vi "New Process.vi"(8 "error in (no error)":errorcluster, 10 "Init options":T1={"UI visible?"=TRUE, "Update rate (ms)"=250, "visible sidebar?"=TRUE, "time to plot (init)"=600.0, "time to plot (max)"=inf, "config file start path"=path ""} {"time to plot (init)" format="%<%H:%M:%S>t"}, 11 "BluePlotHandle in":refnum<class "BluePlotHandle.lvclass">) -> (0 "error out":errorcluster, 2 "VI ref":refnum<vi>, 3 "BluePlotHandle out":refnum<class "BluePlotHandle.lvclass">)   [LabVIEW 2021, in "BluePlot.lvlib" / "BluePlotHandle.lvclass"]
doc: "This will launch a new asynchronous plot instance.\n\n<B>BluePlotHandle in\n</B>This needs to be a user-created object which has dynamic dispatch overrides for satisfying the framework of the package.\n\n<B>Init options</B>\nOptional arguments for affecting the bootup behavior of the plot instance.\nUI Visibile --> Is the UI visible? If no, then the plots are not updated.\nUpdate rate (ms) --> refresh rate of the plots\nvisible sidebar? --> Is the sidebar displaing channel names visible?\ntime to plot (init) --> initial value for the time-to-plot control\ntime to plot (max) --> max allowed entry value for the time-to-plot control\n\n<B>VI ref</B>\nThis output is a reference to the launched plot instance.\nYou are able to insert this into a subpanel, or just open the front panel directly."
uses:
  BluePlotHandle.lvclass
  SubVIs/Init Options.ctl
  TypeDefs/BlueMultiPlot Inputs.ctl
  BluePlot.lvlib
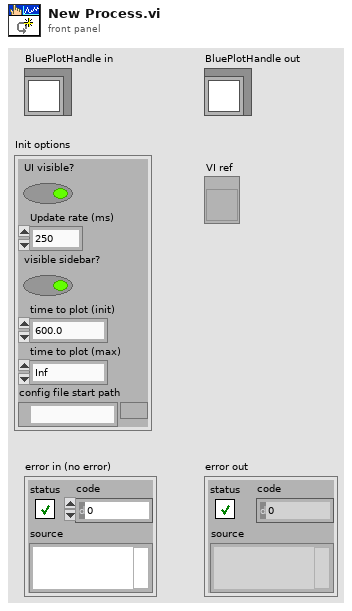
[diagram p1: front panel]
types:
  T1 = typedef "BluePlot.lvlib/BluePlotHandle.lvclass/Init Options.ctl" = cluster{"UI visible?":bool, "Update rate (ms)":u32, "visible sidebar?":bool, "time to plot (init)":dbl, "time to plot (max)":dbl, "config file start path":path}
  T2 = typedef "BluePlot.lvlib/BlueMultiPlot Inputs.ctl" = cluster{"plot menu":string[], "UE: ItemTag":refnum<user-event>}
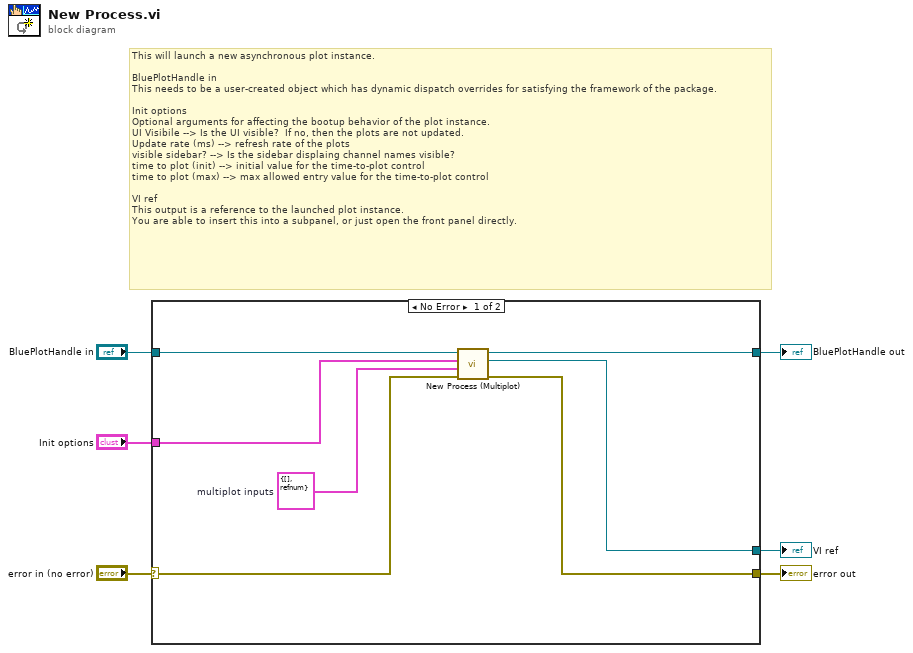
[diagram p0: block diagram]
diagram:
  # "This will launch a new asynchronous plot instance.\n\nBluePlotHandle in\nThis needs to be a user-created object which has dynamic dispatch overrides for satisfying the framework of the package.\n\nInit options\nOptional arguments for affecting the bootup behavior of the plot instance.\nUI Visibile --> Is the UI visible?  If no, then the plots are not updated.\nUpdate rate (ms) --> refresh rate of the plots\nvisible sidebar? --> Is the sidebar displaing channel names visible?\ntime to plot (init) --> initial value for the time-to-plot control\ntime to plot (max) --> max allowed entry value for the time-to-plot control\n\nVI ref\nThis output is a reference to the launched plot instance.\nYou are able to insert this into a subpanel, or just open the front panel directly."
  n1 = case shown="No Error" "error in (no error)" {
    selector: "error in (no error)" -> [w10 w15]
    tunnel: [w11 w15] -> w3
    tunnel: [w12 w14] -> w5
    tunnel: [w8 _] -> w6
    tunnel: "BluePlotHandle in" -> [w13 w14]
    tunnel: "Init options" -> [w9 _]
    frame No Error {
      w7 = T2 {"plot menu"=[], "UE: ItemTag"=refnum}  # multiplot inputs
      n2 = call "New Process (Multiplot).vi"("error in (no error)"=w10, "Multiplot inputs"=w7, "Init options"=w9, "BluePlotHandle in"=w13) -> ("error out"=w11:errorcluster, "VI ref"=w8:refnum<vi>, "BluePlotHandle out"=w12:refnum<class "BluePlotHandle.lvclass">)  [unwired: 5 in]
    }
    frame Error {
    }
  }
  "error out" <- w3
  "BluePlotHandle out" <- w5
  "VI ref" <- w6
